vi "AlliGator Get-Set Phasor Ratio References.vi"(0 "Reference Phasor 1":T1, 1 "Reference Frequency 1":dbl[unit], 5 "Reference Lifetime 1":dbl[unit], 7 "Reference Phasor 2":T1, 9 "Reference Lifetime 2":dbl[unit], 11 "error in (no error)":errorcluster, 12 "Reference Frequency 2":dbl[unit], 13 "Get(F)/Set":bool) -> (2 "All defined?":bool, 3 "Reference Frequency 1":dbl[unit], 4 "Reference Phasor 1":T1, 6 "Reference Lifetime 1":dbl[unit], 8 "Reference Phasor 2":T1, 10 "Reference Lifetime 2":dbl[unit], 14 "Reference Frequency 2":dbl[unit], 15 "error out":errorcluster)   [LabVIEW 2021, in "AlliGator Phasor Ratio.lvlib"]
doc: "Stores the references and their associated data."
uses:
  AlliGator Phasor Ratio.lvlib
  Phasor/Phasor (g, s).ctl
  Globals, Variables, Constants/AlliGator Variables List.ctl
  Globals, Variables, Constants/AlliGator Globals, Variables & Constants.lvlib
  Phasor/Phasor.lvlib
panel:
  # "see the AlliGator License on the block diagram (Ctrl+E or Window:Show Block Diagram)"
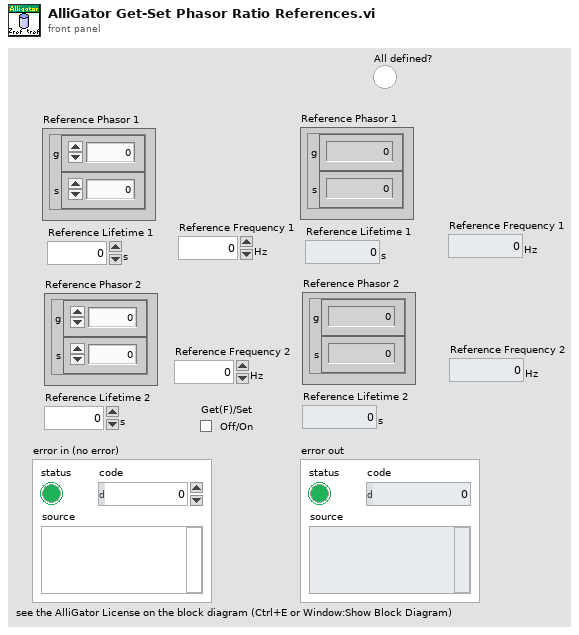
[diagram p1: front panel]
types:
  T1 = typedef "Phasor.lvlib/Phasor (g, s).ctl" = cluster{"g":dbl, "s":dbl}
  T2 = typedef "AlliGator Globals, Variables & Constants.lvlib/AlliGator Variables List.ctl" = enum16{"---- GUI ----", "GUI:Initialization Status", "GUI:State Indicators Refnum", "GUI:Original AlliGator Menu Items", "GUI:Current Action Loop State", "GUI:Script in progress", "GUI:Playback", "GUI:Loop Playback", "GUI:Search ROI Used", "GUI:Search ROI", "Decay Graph Max Legend Size", "Intensity Graph Max Legend Size", "Decay Statistics Graph Max Legend Size", "Phasor Graph Max Legend Size", "Phasor Ratio Graph Max Legend Size", "Lifetime Graph Max Legend Size", "---- Files ----", "Files:Export Dataset Frames as Individual Files", "Files:Show Batch Export Help Balloons", "Files:Frames in Dataset", "Files:ptu File Frame Start Indices", "Files:Current Frame in Dataset", "Files:Current Frame Timestamp", "Files:Dataset Loaded", "Files:Dataset Metadata", "Files:Dataset Channel", "Files:Dataset Data Description", "Files:Background Dataset Metadata", "Files:Background Dataset Channel", "Files:Background Dataset Data Description", "Files:Background File Subtraction", "Files:Background File Path", "Files:Background File Pile-up Correction", "Files:Background File Pixel Well Capacity", "Files:Background File Scaling Factor", "Files:Current Dataset Load Settings", "Files:Dataset Path", "Files:ICCD-specific Information", "Files:Macrotime Gate Separation", "------ Python Plugins ------", "Python Plugins:Information", "Python Plugins:Python Session", "Python Plugins:Valid Python Session?", "---- Source Image ----", "Source Image:ROIs", "Source Image:Current ROI", "Source Image:ROI Event Refnum", "X_Source Image Display Range", "X_Source Image Palette Information", "X_Type of Displayed Image", "X_Time Gate Slider", "Source Image:Palette List", "Source Image:Scale", "Source Image:ROI Overlay Color", "Source Image:Overlay to Erase", "Source Image:Is Displayed Image Accumulated", "Source Image:White Light Image Modified", "Source Image:Mask Image Modified", "---- Image Profile Window ----", "Image Profile:Window Event Refnum", "Image Profile:IntensityType", "Image Profile:Intensity Average Type", "Image Profile:Intensity-weighted SDV", "Image Profile:Box Profile Type", "Image Profile:Window Open", "Image Profile:Plotted Fit Parameter", "------ Phasor Graph -------", "Phasor Graph:Show Line", "---- Phasor Plot ---", "Phasor Plot:Parameters Changed", "Phasor Plot:FLI Dataset Modified since last Calculation", "Phasor Harmonics Data", "Selected Phasor Harmonics", "Phasor Harmonic Manager Event Refnum", "Phasor Plot:ROIs", "Phasor Plot:Current ROI", "Phasor Plot:ROI Event Refnum", "Phasor Plot:Image Reference Points", "Phasor Plot:Computed", "Phasor Plot:Palette Information", "Phasor Plot:Palette List", "Phasor Plot:Phasor Ratio Palette Information", "Phasor Plot:Phasor Ratio Palette List", "Phasor Plot:Image Scale", "Phasor Plot:Image Overlay to Erase", "Phasor Plot:Image Elements to Update", "Phasor Plot:Current Calculation Parameters", "Phasor Plot:Current Calibration Options", "Phasor Plot:Reset Cumulated Phasor Plot", "Phasor Plot:Reference 1", "Phasor Plot:Lifetime Reference 1", "Phasor Plot:Reference 1 Frequency", "Phasor Plot:Reference 2", "Phasor Plot:Lifetime Reference 2", "Phasor Plot:Reference 2 Frequency", "---- Decay Analysis ----", "Number of Selected Decays to Fit", "LS Fit Results", "LAR Fit Results", "BS Fit Results", "Last Decay Max - Min", "Best Fit Parameters", "Best Fit Parameter Names", "Actual Size X", "Actual Size Y", "Binning X", "Binning Y", "Actual # Gates", "Dataset Number", "Gates to...", "Gates Skipped", "Gates to keep", "Gate Step", "Gate Separation", "Reversed Gates", "Pile-up Correction", "Pixel Well Capacity", "Background Subtracted", "Background Subtraction Method", "Background Definition Range", "Background File (deprecated)", "Number of Dataset Accumulated", "Array of Accumulated Dataset Paths", "Do Averaged Datasets", "Destination File Path", "Process Plot Target", "Use 1/D as Phasor Frequency", "---- Decay Fit Parameter Map -----", "Decay Fit Parameter Map:Palette Information", "Decay Fit Parameter Map:Palette List", "---- Parameter Map ----", "Parameter Map:Palette Information", "Parameter Map:Palette List", "------- Local Decay Window ---------", "Local Decay Graph Window:Event Refnum", "Local Decay Graph Window:Use normalized IRF for convolution", "----- Miscellaneous ----", "Misc:Skippable Dialog Windows Status"}
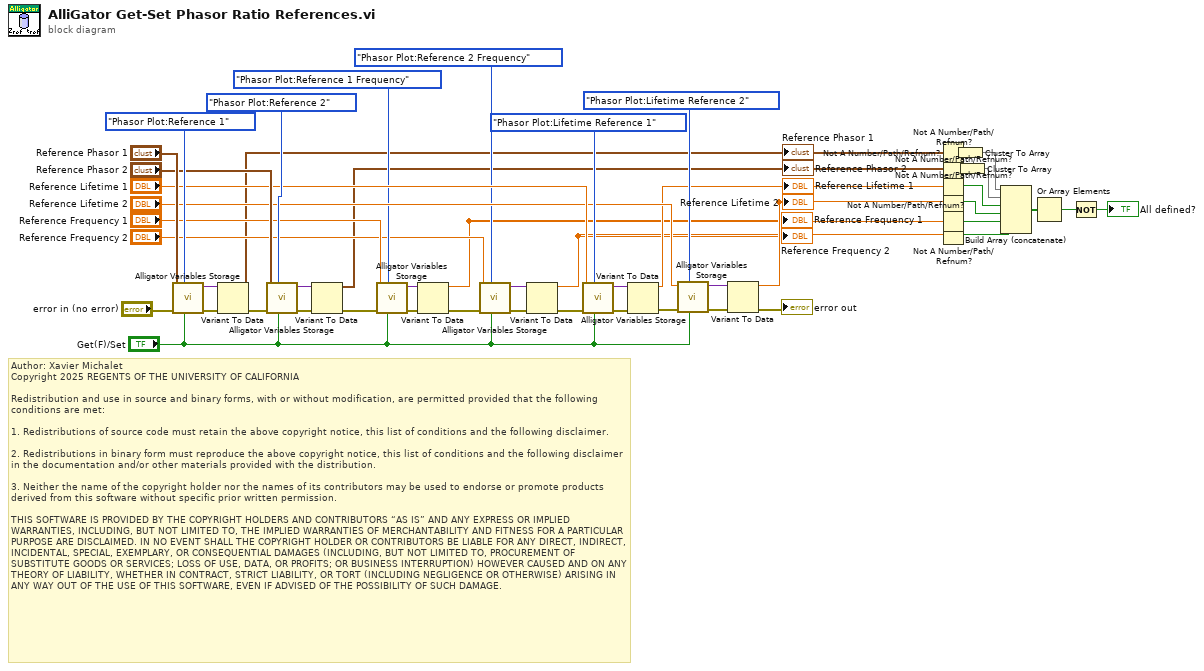
[diagram p0: block diagram]
diagram:
  # "Author: Xavier Michalet\nCopyright 2025 REGENTS OF THE UNIVERSITY OF CALIFORNIA\n\nRedistribution and use in source and binary forms, with or without modification, are permitted provided that the following conditions are met:\n\n1. Redistributions of source code must retain the above copyright notice, this list of conditions and the following disclaimer.\n\n2. Redistributions in binary form must reproduce the above copyright notice, this list of conditions and the following disclaimer in the documentation and/or other materials provided with the distribution.\n\n3. Neither the name of the copyright holder nor the names of its contributors may be used to endorse or promote products derived from this software without specific prior written permission.\n\nTHIS SOFTWARE IS PROVIDED BY THE COPYRIGHT HOLDERS AND CONTRIBUTORS “AS IS” AND ANY EXPRESS OR IMPLIED WARRANTIES, INCLUDING, BUT NOT LIMITED TO, THE IMPLIED WARRANTIES OF MERCHANTABILITY AND FITNESS FOR A PARTICULAR PURPOSE ARE DISCLAIMED. IN NO EVENT SHALL THE COPYRIGHT HOLDER OR CONTRIBUTORS BE LIABLE FOR ANY DIRECT, INDIRECT, INCIDENTAL, SPECIAL, EXEMPLARY, OR CONSEQUENTIAL DAMAGES (INCLUDING, BUT NOT LIMITED TO, PROCUREMENT OF SUBSTITUTE GOODS OR SERVICES; LOSS OF USE, DATA, OR PROFITS; OR BUSINESS INTERRUPTION) HOWEVER CAUSED AND ON ANY THEORY OF LIABILITY, WHETHER IN CONTRACT, STRICT LIABILITY, OR TORT (INCLUDING NEGLIGENCE OR OTHERWISE) ARISING IN ANY WAY OUT OF THE USE OF THIS SOFTWARE, EVEN IF ADVISED OF THE POSSIBILITY OF SUCH DAMAGE."
  n1 = call "Alligator Variables Storage.vi"("Get(F)/Set"="Get(F)/Set", "AlliGator Variable"=AlliGator_Variables_List."Phasor Plot:Reference 1" ("Alligator Variable"), "Error In"="error in (no error)", "Data in"="Reference Phasor 1") -> ("Error Out"=w42:errorcluster, "Data out"=w44:variant)  [unwired: 5 in, 1 out]
  n2 = Variant To Data(error in=w42, Variant=w44) -> (data=w17:T1, error out=w45:errorcluster)  [unwired: 1 in]
  "Reference Phasor 1" <- w17
  n3 = call "Alligator Variables Storage.vi"("Get(F)/Set"="Get(F)/Set", "AlliGator Variable"=AlliGator_Variables_List."Phasor Plot:Reference 2" ("Alligator Variable"), "Error In"=w45, "Data in"="Reference Phasor 2") -> ("Error Out"=w47:errorcluster, "Data out"=w41:variant)  [unwired: 5 in, 1 out]
  n4 = Variant To Data(error in=w47, Variant=w41) -> (data=w16:T1, error out=w29:errorcluster)  [unwired: 1 in]
  "Reference Phasor 2" <- w16
  n5 = call "Alligator Variables Storage.vi"("Get(F)/Set"="Get(F)/Set", "AlliGator Variable"=AlliGator_Variables_List."Phasor Plot:Reference 1 Frequency" ("Alligator Variable"), "Error In"=w29, "Data in"="Reference Frequency 1") -> ("Error Out"=w27:errorcluster, "Data out"=w26:variant)  [unwired: 5 in, 1 out]
  n6 = Variant To Data(error in=w27, Variant=w26) -> (data=w13:dbl[unit], error out=w25:errorcluster)  [unwired: 1 in]
  "Reference Frequency 1" <- w13
  n7 = call "Alligator Variables Storage.vi"("Get(F)/Set"="Get(F)/Set", "AlliGator Variable"=AlliGator_Variables_List."Phasor Plot:Reference 2 Frequency" ("Alligator Variable"), "Error In"=w25, "Data in"="Reference Frequency 2") -> ("Error Out"=w24:errorcluster, "Data out"=w22:variant)  [unwired: 5 in, 1 out]
  n8 = Variant To Data(error in=w24, Variant=w22) -> (data=w12:dbl[unit], error out=w23:errorcluster)  [unwired: 1 in]
  "Reference Frequency 2" <- w12
  n9 = call "Alligator Variables Storage.vi"("Get(F)/Set"="Get(F)/Set", "AlliGator Variable"=AlliGator_Variables_List."Phasor Plot:Lifetime Reference 1" ("Alligator Variable"), "Error In"=w23, "Data in"="Reference Lifetime 1") -> ("Error Out"=w35:errorcluster, "Data out"=w36:variant)  [unwired: 5 in, 1 out]
  n10 = Variant To Data(error in=w35, Variant=w36) -> (data=w15:dbl[unit], error out=w37:errorcluster)  [unwired: 1 in]
  "Reference Lifetime 1" <- w15
  n11 = call "Alligator Variables Storage.vi"("Get(F)/Set"="Get(F)/Set", "AlliGator Variable"=AlliGator_Variables_List."Phasor Plot:Lifetime Reference 2" ("Alligator Variable"), "Error In"=w37, "Data in"="Reference Lifetime 2") -> ("Error Out"=w38:errorcluster, "Data out"=w39:variant)  [unwired: 5 in, 1 out]
  n12 = Variant To Data(error in=w38, Variant=w39) -> (data=w14:dbl[unit], error out=→"error out":errorcluster)  [unwired: 1 in]
  "Reference Lifetime 2" <- w14
  n13 = Not A Number/Path/Refnum?(number/path/refnum=w17) -> (NaN/Path/Refnum?=w6:cluster{"g":bool, "s":bool})
  n14 = Not A Number/Path/Refnum?(number/path/refnum=w16) -> (NaN/Path/Refnum?=w7:cluster{"g":bool, "s":bool})
  n15 = Not A Number/Path/Refnum?(number/path/refnum=w15) -> (NaN/Path/Refnum?=w8:bool)
  n16 = Not A Number/Path/Refnum?(number/path/refnum=w14) -> (NaN/Path/Refnum?=w9:bool)
  n17 = Not A Number/Path/Refnum?(number/path/refnum=w13) -> (NaN/Path/Refnum?=w10:bool)
  n18 = Not A Number/Path/Refnum?(number/path/refnum=w12) -> (NaN/Path/Refnum?=w11:bool)
  n19 = Cluster To Array(cluster=w6) -> (array=w4:bool[])
  n20 = Cluster To Array(cluster=w7) -> (array=w5:bool[])
  n21 = Build Array (concatenate)(w4, w5, w8, w9, w10, w11) -> (w3:bool[])
  n22 = Or Array Elements(Boolean array=w3) -> (logical OR=w2:bool)
  n23 = Not(x=w2) -> (.not. x?=→"All defined?":bool)
